vi "sensor get monitor type.vi"(10 "dest":u32(ring) items=["MONITOR_OPAL", "MONITOR_EMERALD", "MONITOR_SAPHIRE"], 11 "case_id_string":string) -> (2 "dest out":u32(ring) items=["MONITOR_OPAL", "MONITOR_EMERALD", "MONITOR_SAPHIRE"], 3 "function return":i32)   [LabVIEW 2019, in "apdm.lvlib"]
doc: "APDM_EXPORT int apdm_sensor_get_monitor_type(const char *case_id_string, apdm_monitor_type_t *dest);"
uses:
  apdm.lvlib
  Lee Lab/CP FES Walking 2018/Code/Working/LabVIEW/apdm.dll
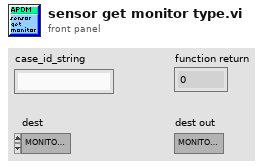
[diagram p1: front panel]
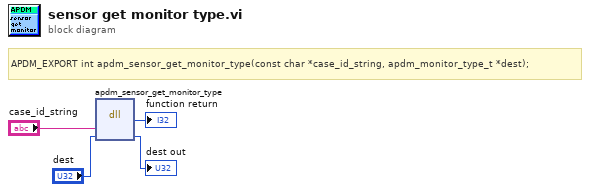
[diagram p0: block diagram]
diagram:
  # "APDM_EXPORT int apdm_sensor_get_monitor_type(const char *case_id_string, apdm_monitor_type_t *dest);"
  n1 = dll-call lib="C:/Users/jfalesi/Dropbox/Lee Lab/CP FES Walking 2018/Code/Working/LabVIEW/apdm.*" fn="apdm_sensor_get_monitor_type"("case_id_string"="case_id_string", "dest"="dest") -> (→"function return":i32, "dest"=→"dest out":u32)  [unwired: 4 in, 2 out]
